vi "Python Escape Codes.vi"() -> (0 "Python Escape Codes":T1(array[cluster]))   [LabVIEW 2020, in "jki_python_data_tools.lvlib"]
uses:
  jki_python_data_tools.lvlib
panel:
  # "Copyright © 2003-2009 JKI. All rights reserved.\n\nAuthor: Jim Kring [jim.kring@jameskring.com]\n\nThis library is provided \"AS IS\" ,WITHOUT WARRANTIES OR \nCONDITIONS OF ANY KIND, either express or implied.\n\nJames Kring, Inc. -- http://www.jameskring.com"
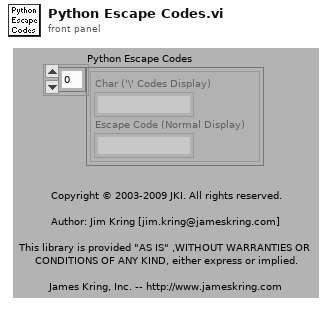
[diagram p1: front panel]
types:
  T1 = cluster{"Char ('\\' Codes Display)":string, "Escape Code (Normal Display)":string}[]
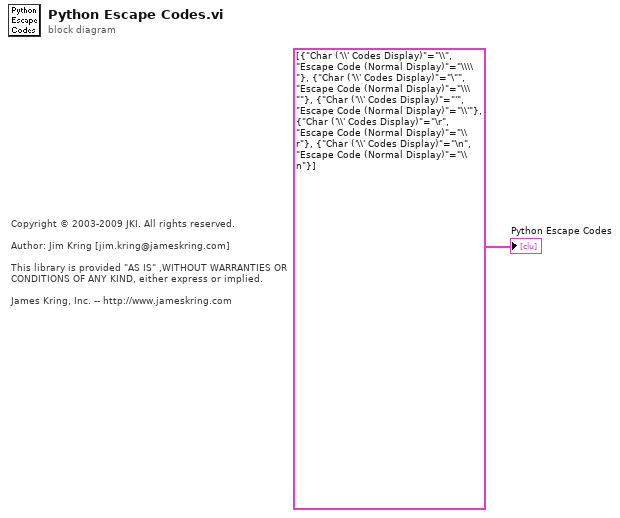
[diagram p0: block diagram]
diagram:
  # "Copyright © 2003-2009 JKI. All rights reserved.\n\nAuthor: Jim Kring [jim.kring@jameskring.com]\n\nThis library is provided \"AS IS\" ,WITHOUT WARRANTIES OR \nCONDITIONS OF ANY KIND, either express or implied.\n\nJames Kring, Inc. -- http://www.jameskring.com"
  "Python Escape Codes" <- T1 [{"Char ('\\' Codes Display)"="\\", "Escape Code (Normal Display)"="\\\\"}, {"Char ('\\' Codes Display)"="\"", "Escape Code (Normal Display)"="\\\""}, {"Char ('\\' Codes Display)"="'", "Escape Code (Normal Display)"="\\'"}, {"Char ('\\' Codes Display)"="\r", "Escape Code (Normal Display)"="\\r"}, {"Char ('\\' Codes Display)"="\n", "Escape Code (Normal Display)"="\\n"}]
